vi "Get Text Size.vi"(6 "Thickness (Default: 1)":i32=1, 7 "Text Drawing Settings (Default: Simplex)":T2={"OpenCV Font Face"=enum."FONT_HERSHEY_SIMPLEX", "Font Scale"=1.0}, 8 "error in (no error)":errorcluster, 11 "Text":string) -> (0 "error out":errorcluster, 1 "Base Line":i32, 3 "Size":T1)   [LabVIEW 2020, in "g_ar_toolkit.image.lvlib"]
uses:
  g_ar_toolkit.image.lvlib
  Text Drawing Settings.ctl
  Font Face.ctl
  g_ar_toolkit.common/Image Size (Integer).ctl
  g_ar_toolkit.common/g_ar_toolkit.common.lvlib
  bin/g_ar_toolkit.1.32.dll
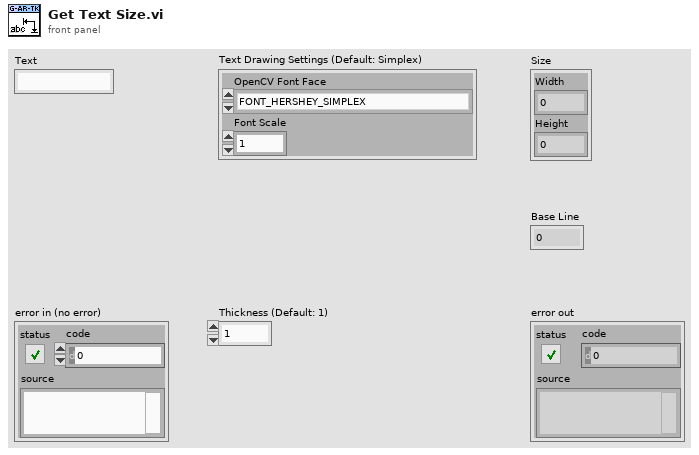
[diagram p1: front panel]
types:
  T1 = typedef "g_ar_toolkit.common.lvlib/Image Size (Integer).ctl" = cluster{"Width":u16, "Height":u16}
  T2 = typedef "g_ar_toolkit.image.lvlib/Text Drawing Settings.ctl" = cluster{"OpenCV Font Face":T3, "Font Scale":dbl}
  T3 = typedef "g_ar_toolkit.image.lvlib/Font Face.ctl" = enum16{"FONT_HERSHEY_SIMPLEX", "FONT_HERSHEY_PLAIN", "FONT_HERSHEY_DUPLEX", "FONT_HERSHEY_COMPLEX", "FONT_HERSHEY_TRIPLEX", "FONT_HERSHEY_COMPLEX_SMALL", "FONT_HERSHEY_SCRIPT_SIMPLEX", "FONT_HERSHEY_SCRIPT_COMPLEX", "FONT_ITALIC"}
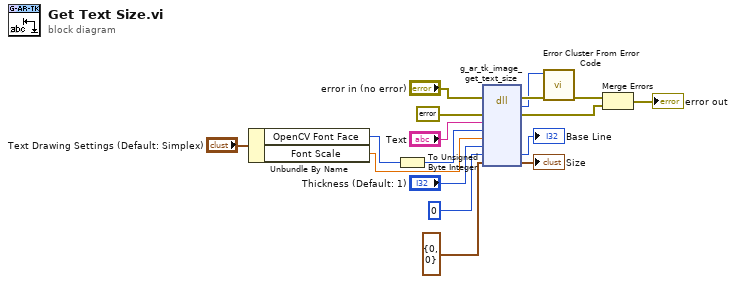
[diagram p0: block diagram]
diagram:
  n1 = Unbundle By Name("Text Drawing Settings (Default: Simplex)") -> ("OpenCV Font Face"=w10:T3, "Font Scale"=w12:dbl)
  n2 = To Unsigned Byte Integer(number=w10) -> (unsigned 8bit integer=w11:u8)
  n3 = dll-call lib="C:/serenial/libraries/g-augmented-reality-toolkit/LabVIEW/bin/g_ar_toolkit.1.*.*" fn="g_ar_tk_image_get_text_size"(error in="error in (no error)", "error_cluster"=errorcluster {"status"=FALSE, "code"=0, "source"=""} ("error constant"), "text"="Text", "font_face"=w11, "font_scale"=w12, "thickness"="Thickness (Default: 1)", "base_line"=0, "size"=T1 {"Width"=0, "Height"=0} ("Size")) -> (error out=w9:errorcluster, "MgErr"=w8:i32, "error_cluster"=w5:errorcluster, "base_line"=→"Base Line":i32, "size"=→"Size":T1)  [unwired: 6 in, 1 out]
  n4 = call <vilib>:"Error Cluster From Error Code.vi"("error in (no error)"=w9, "error code (0)"=w8) -> ("error out"=w7:errorcluster)  [unwired: 7 in]
  n5 = Merge Errors(w7, w5) -> (→"error out":errorcluster)
